vi "Get Templates.vi"(8 "error in (no error)":errorcluster, 11 "eLab in":refnum<class "PL eLabFTW Client.lvclass">) -> (0 "error out":errorcluster, 2 "templates":T1(array[cluster]) {"lock"."datetime" format="%<%X\n%x>T"}, 3 "eLab out":refnum<class "PL eLabFTW Client.lvclass">)   [LabVIEW 2015, in "PL eLabFTW Client.lvclass"]
doc: "Gets templates."
uses:
  PL eLabFTW Client.lvclass
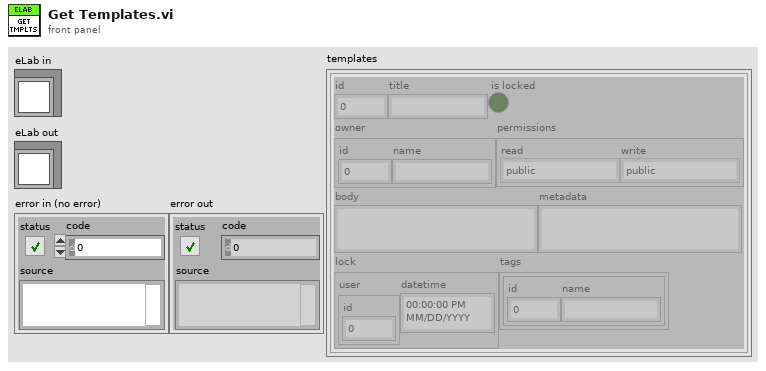
[diagram p1: front panel]
types:
  T1 = cluster{"id":u32, "title":string, "is locked":bool, "owner":cluster{"id":u32, "name":string}, "permissions":cluster{"read":enum16{"public", "organization", "team", "owner and admins", "owner"}, "write":enum16{"public", "organization", "team", "owner and admins", "owner"}}, "body":string, "metadata":string, "lock":cluster{"user":cluster{"id":u32}, "datetime":timestamp}, "tags":cluster{"id":u32, "name":string}[]}[]
  T2 = cluster{"id":string, "title":string, "body":string, "userid":string, "canread":string, "canwrite":string, "locked":string, "lockedby":string, "lockedwhen":string, "fullname":string, "metadata":string, "teams_id":string, "tags":string, "tags_id":string}[]
  T3 = cluster{"id":u32, "title":string, "is locked":bool, "owner":cluster{"id":u32, "name":string}, "permissions":cluster{"read":enum16{"public", "organization", "team", "owner and admins", "owner"}, "write":enum16{"public", "organization", "team", "owner and admins", "owner"}}, "body":string, "metadata":string, "lock":cluster{"user":cluster{"id":u32}, "datetime":timestamp}, "tags":cluster{"id":u32, "name":string}[]}
  T4 = enum16{"public", "organization", "team", "owner and admins", "owner"}
  T5 = cluster{"id":i32, "title":i32, "body":i32, "userid":i32, "canread":i32, "canwrite":i32, "locked":i32, "lockedby":i32, "lockedwhen":i32, "fullname":i32, "metadata":i32, "teams_id":i32, "tags":i32, "tags_id":i32}
  T6 = cluster{"id":bool, "title":bool, "body":bool, "userid":bool, "canread":bool, "canwrite":bool, "locked":bool, "lockedby":bool, "lockedwhen":bool, "fullname":bool, "metadata":bool, "teams_id":bool, "tags":bool, "tags_id":bool}
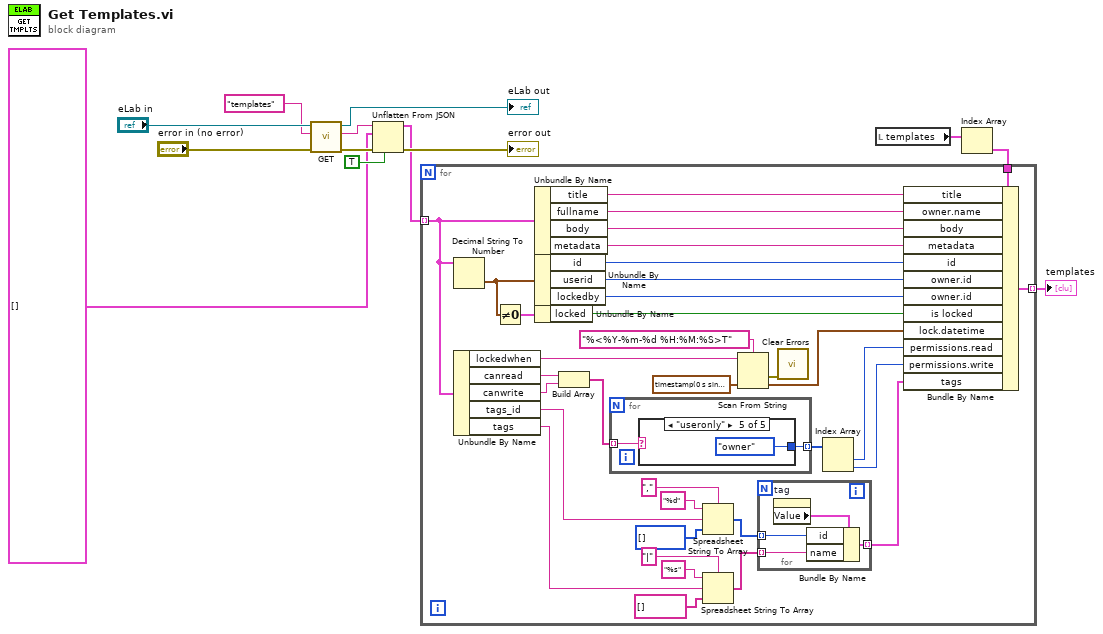
[diagram p0: block diagram]
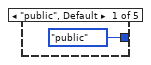
[diagram p2: hidden frame]
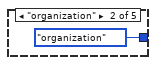
[diagram p3: hidden frame]
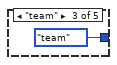
[diagram p4: hidden frame]
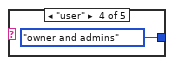
[diagram p5: hidden frame]
diagram:
  n1 = call "GET.vi"("error in (no error)"="error in (no error)", "relative URL"="templates" ("format string"), "eLab in"="eLab in") -> ("error out"=w10:errorcluster, "response body"=w6:string, "eLab out"=→"eLab out":refnum<class "PL eLabFTW Client.lvclass">)  [unwired: 6 in]
  n2 = Unflatten From JSON(JSON string=w6, type and defaults=T2 [], default null elements? (F)=TRUE, error in (no error)=w10) -> (value=w7:T2, error out=→"error out":errorcluster)  [unwired: 3 in]
  n3 = local read "templates"() -> (w4:T1)
  n4 = Index Array(array=w4) -> (element=w3:T3)  [unwired: 1 in]
  n5 = for {
    tunnel: w7 -> [w33] mode=indexing
    tunnel: w3 -> [w15]
    tunnel: [w14] -> w2 mode=indexing
    n6 = Decimal String To Number(string=w33) -> (number=w44:T5)  [unwired: 2 in, 1 out]
    n7 = Unbundle By Name(w33) -> ("lockedwhen"=w20:string, "canread"=w41:string, "canwrite"=w40:string, "tags_id"=w26:string, "tags"=w25:string)
    n8 = Not Equal To 0?(x=w44) -> (x != 0?=w43:T6)
    n9 = Unbundle By Name(w33) -> ("title"=w48:string, "fullname"=w47:string, "body"=w36:string, "metadata"=w35:string)
    n10 = Unbundle By Name(w44) -> ("id"=w46:i32, "userid"=w45:i32, "lockedby"=w34:i32)
    n11 = Unbundle By Name(w43) -> ("locked"=w42:bool)
    n12 = Build Array(w41, w40) -> (w39:string[])
    n13 = for {
      tunnel: w39 -> [w54] mode=indexing
      tunnel: [w53] -> w38 mode=indexing
      n14 = case shown="\"useronly\"" w54 {
        tunnel: [T4."public" ("permissions.read") T4."organization" ("permissions.read") T4."team" ("permissions.read") T4."owner and admins" ("permissions.read") T4."owner" ("permissions.read")] -> w53
        frame "public", Default {
        }
        frame "organization" {
        }
        frame "team" {
        }
        frame "user" {
        }
        frame "useronly" {
        }
      }
    }
    n15 = Spreadsheet String To Array(delimiter (Tab)=",", format string="%d", spreadsheet string=w26, array type (2D Dbl)=u32[] []) -> (array=w24:u32[])
    n16 = Spreadsheet String To Array(delimiter (Tab)="|", format string="%s", spreadsheet string=w25, array type (2D Dbl)=string[] []) -> (array=w23:string[])
    n17 = Scan From String(format string="%<%Y-%m-%d %H:%M:%S>T", input string=w20, default 1=timestamp(0 s since 1904-01-01) ("from")) -> (error out=w22:errorcluster, output 1=w19:timestamp)  [unwired: 2 in, 2 out]
    n18 = for {
      tunnel: [w51] -> w16 mode=indexing
      tunnel: w24 -> [w50] mode=indexing
      tunnel: w23 -> [w49] mode=indexing
      n19 = property on="tag" class="Clust (strict)"() -> ("Value"=w52:cluster{"id":u32, "name":string})  [unwired: 2 in, 2 out]
      n20 = Bundle By Name(cluster=w52, "id"=w50, "name"=w49) -> (w51:cluster{"id":u32, "name":string})
    }
    n21 = call <vilib>:"Clear Errors.vi"("error in (no error)"=w22) -> ()  [unwired: 5 in, 2 out]
    n22 = Index Array(array=w38) -> (element #1=w18:T4, element #2=w17:T4)  [unwired: 2 in]
    n23 = Bundle By Name(cluster=w15, "title"=w48, "owner.name"=w47, "body"=w36, "metadata"=w35, "id"=w46, "owner.id"=w45, "owner.id"=w34, "is locked"=w42, "lock.datetime"=w19, "permissions.read"=w18, "permissions.write"=w17, "tags"=w16) -> (w14:T3)
  }
  "templates" <- w2
